vi "Disconnect.vi"(8 "error in (no error)":errorcluster, 11 "VISA resource name":refnum<visa-resource-name>) -> (0 "error out":errorcluster, 3 "VISA resource name out":refnum<visa-resource-name>)   [LabVIEW 2019, in "Mark 10 TSTM-DC.lvlib"]
uses:
  Mark 10 TSTM-DC.lvlib
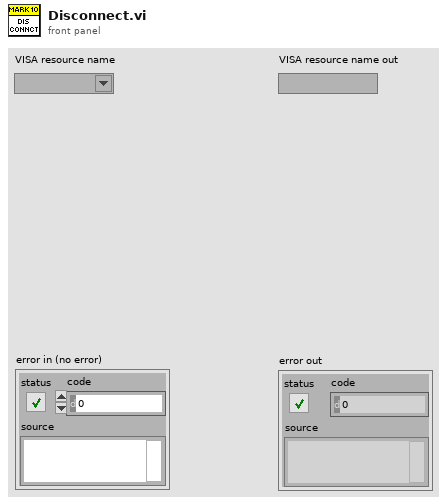
[diagram p1: front panel]
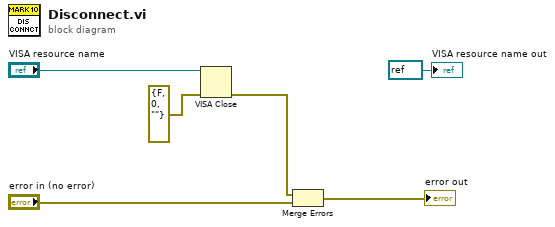
[diagram p0: block diagram]
diagram:
  n1 = VISA Close(VISA resource name="VISA resource name", error in (no error)=errorcluster {"status"=FALSE, "code"=0, "source"=""}) -> (error out=w2:errorcluster)
  n2 = Merge Errors(w2, "error in (no error)") -> (→"error out":errorcluster)
  "VISA resource name out" <- refnum<visa-resource-name> refnum ("VISA resource name out")
